vi "runMonoExecuter.vi"(8 "error in (no error)":errorcluster, 11 "MonoCommunicator in":refnum<class "MonoCommunicator.lvclass">) -> (0 "error out":errorcluster, 3 "MonoCommunicator out":refnum<class "MonoCommunicator.lvclass">)   [LabVIEW 2016, in "MonoCommunicator.lvclass"]
uses:
  MonoCommunicator.lvclass
  MonoCommunicator.lvclass/MonoCommunicator.ctl
  CommandParser/CommandParser.lvclass
  Typedefs/slit.ctl
  Typedefs/SlitType.ctl
  Typedefs/slitWidth.ctl
  MonoPubSubData/MonoPubSubData.lvclass
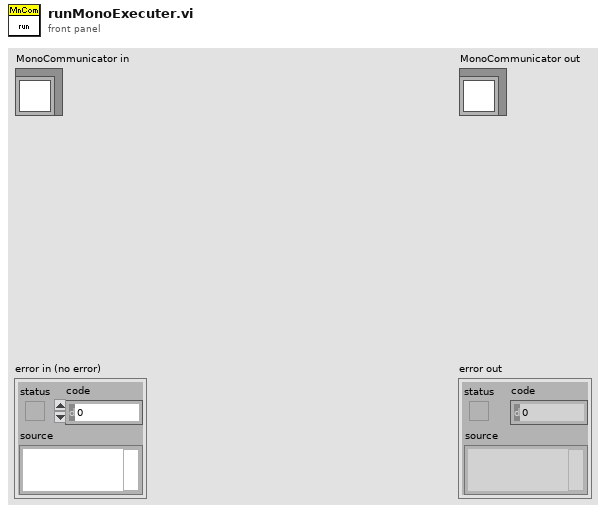
[diagram p1: front panel]
types:
  T1 = cluster{"publishersRegs":refnum<event-registration>, "stopRegs":refnum<event-registration>, "msgReceivedEvent":refnum<event-registration>}
  T2 = typedef "slit.ctl" = cluster{"SlitType":T3, "Width":T4}
  T3 = typedef "SlitType.ctl" = enum16{"Front Entrance", "Side Entrance", "Front Exit", "Side Exit", "First Intermediate", "Second Intermediate"}
  T4 = typedef "slitWidth.ctl" = dbl
  T5 = typedef "MonoCommand.ctl" = enum16{"getGrating", "getFrontEntranceSlitPosition", "getFrontExitSlitPosition", "getWavelength", "setWavelength", "setGrating", "setFrontEntranceSlitPosition", "setFrontExitSlitPosition", "calibrateWavelength", "getStatus", "Unknown", "reset"}
  T6 = typedef "wavelength.ctl" = dbl
  T7 = typedef "DeviceStatus.ctl" = enum16{"SettingUp", "Ready", "Offline", "Fault"}
  T8 = typedef "GratingType.ctl" = enum16{"NoGrating", "Red", "Blue", "Mirror"}
  T9 = typedef "slitPosition.ctl" = dbl
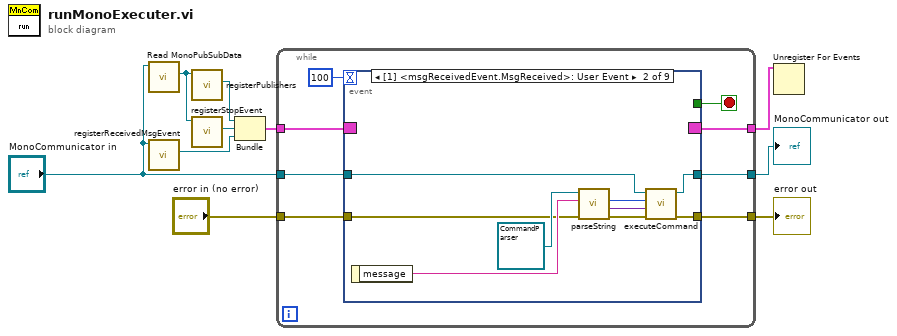
[diagram p0: block diagram]
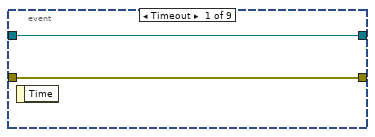
[diagram p2: hidden frame]
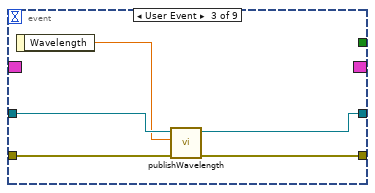
[diagram p3: hidden frame]
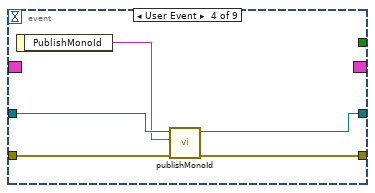
[diagram p4: hidden frame]
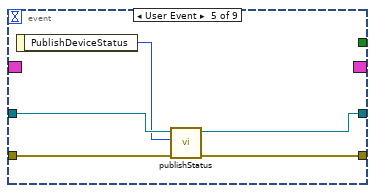
[diagram p5: hidden frame]
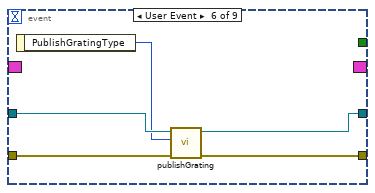
[diagram p6: hidden frame]
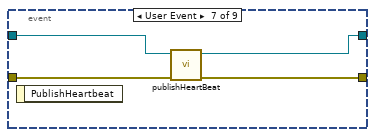
[diagram p7: hidden frame]
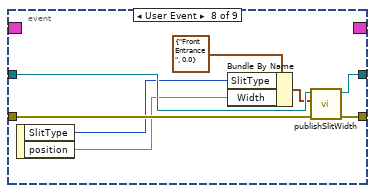
[diagram p8: hidden frame]
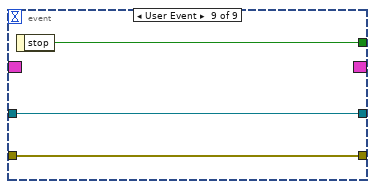
[diagram p9: hidden frame]
diagram:
  n1 = call "Read MonoPubSubData.vi"("MonoCommunicator in"="MonoCommunicator in") -> ("MonoPubSubData.lvclass"=w8:refnum<class "MonoPubSubData.lvclass">)  [unwired: 8 in, 2 out]
  n2 = call "registerReceivedMsgEvent.vi"("MonoCommunicator in"="MonoCommunicator in") -> ("msgReceivedEvent"=w1:refnum<event-registration>)  [unwired: 8 in, 2 out]
  n3 = call "registerPublishers.vi"("MonoPubSubData in"=w8) -> ("publishersRegs"=w6:refnum<event-registration>)  [unwired: 8 in, 2 out]
  n4 = call "registerStopEvent.vi"("MonoPubSubData in"=w8) -> ("stopRegs"=w7:refnum<event-registration>)  [unwired: 8 in, 2 out]
  n5 = Bundle("publishersRegs"=w6, "stopRegs"=w7, "msgReceivedEvent"=w1) -> (w5:T1)  [unwired: 1 in]
  n6 = while {
    tunnel: "error in (no error)" -> [w13]
    tunnel: "MonoCommunicator in" -> [w14]
    tunnel: [w17] -> w9
    tunnel: w5 -> [w16]
    tunnel: [w12] -> w4
    tunnel: [w11] -> w3
    stop <- w15 stop-if-true
    n7 = event shown="[1] <msgReceivedEvent.MsgReceived>: User Event" {
      selector: w16 -> [_ _ _ _ _ _ _ _ _]
      dyn-events: [_ _ _ _ _ _ _ _ _] -> w17
      timeout: 100 -> [_ _ _ _ _ _ _ _ _]
      tunnel: [_ _ _ _ _ _ _ _ w64] -> w15
      tunnel: w14 -> [w19 w23 w34 w38 w43 w47 w52 w59 w63]
      tunnel: w13 -> [w20 w27 w32 w39 w41 w46 w53 w58 w62]
      tunnel: [w20 w25 w31 w36 w40 w49 w50 w61 w62] -> w12
      tunnel: [w19 w24 w30 w35 w44 w48 w51 w60 w63] -> w11
      event Timeout {
        n8 = event-data() -> ()  [unwired: 1 in, 1 out]
      }
      event User Event {
        n9 = event-data() -> ("message"=w28:string)  [unwired: 1 in]
        n10 = call "parseString.vi"("error in (no error)"=w27, "stringCommand"=w28, "CommandParser in"=refnum<class "CommandParser.lvclass"> refnum ("CommandParser.lvclass")) -> ("error out"=w26:errorcluster, "parameter"=w21:variant, "monoCommand"=w22:T5)  [unwired: 5 in, 1 out]
        n11 = call "executeCommand.vi"("error in (no error)"=w26, "parameter"=w21, "monoCommand"=w22, "MonoCommunicator in"=w23) -> ("error out"=w25:errorcluster, "MonoCommunicator out"=w24:refnum<class "MonoCommunicator.lvclass">)  [unwired: 6 in]
      }
      event User Event {
        n12 = event-data() -> ("Wavelength"=w33:T6)  [unwired: 1 in]
        n13 = call "publishWavelength.vi"("error in (no error)"=w32, "wavelength"=w33, "MonoCommunicator in"=w34) -> ("error out"=w31:errorcluster, "MonoCommunicator out"=w30:refnum<class "MonoCommunicator.lvclass">)  [unwired: 7 in]
      }
      event User Event {
        n14 = event-data() -> ("PublishMonoId"=w37:string)  [unwired: 1 in]
        n15 = call "publishMonoId.vi"("error in (no error)"=w39, "monoId"=w37, "MonoCommunicator in"=w38) -> ("error out"=w36:errorcluster, "MonoCommunicator out"=w35:refnum<class "MonoCommunicator.lvclass">)  [unwired: 7 in]
      }
      event User Event {
        n16 = event-data() -> ("PublishDeviceStatus"=w42:T7)  [unwired: 1 in]
        n17 = call "publishStatus.vi"("error in (no error)"=w41, "DeviceStatus"=w42, "MonoCommunicator in"=w43) -> ("error out"=w40:errorcluster, "MonoCommunicator out"=w44:refnum<class "MonoCommunicator.lvclass">)  [unwired: 7 in]
      }
      event User Event {
        n18 = event-data() -> ("PublishGratingType"=w45:T8)  [unwired: 1 in]
        n19 = call "publishGrating.vi"("error in (no error)"=w46, "GratingType"=w45, "MonoCommunicator in"=w47) -> ("error out"=w49:errorcluster, "MonoCommunicator out"=w48:refnum<class "MonoCommunicator.lvclass">)  [unwired: 7 in]
      }
      event User Event {
        n20 = event-data() -> ()  [unwired: 1 in, 1 out]
        n21 = call "publishHeartBeat.vi"("error in (no error)"=w53, "MonoCommunicator in"=w52) -> ("error out"=w50:errorcluster, "MonoCommunicator out"=w51:refnum<class "MonoCommunicator.lvclass">)  [unwired: 8 in]
      }
      event User Event {
        n22 = event-data() -> ("SlitType"=w57:T3, "position"=w56:T9)  [unwired: 1 in]
        n23 = Bundle By Name(cluster=T2 {"SlitType"=enum."Front Entrance", "Width"=0.0} ("slitPosition"), "SlitType"=w57, "Width"=w56) -> (w55:T2)
        n24 = call "publishSlitWidth.vi"("error in (no error)"=w58, "position"=w55, "MonoCommunicator in"=w59) -> ("error out"=w61:errorcluster, "MonoCommunicator out"=w60:refnum<class "MonoCommunicator.lvclass">)  [unwired: 7 in]
      }
      event User Event {
        n25 = event-data() -> ("stop"=w64:bool)  [unwired: 1 in]
      }
    }
  }
  "error out" <- w4
  "MonoCommunicator out" <- w3
  n26 = Unregister For Events(event registration refnum=w9) -> ()  [unwired: 1 in, 1 out]
